vi "Constructor.vi"(11 "Graph Reference":refnum<vi>) -> (3 "Graph Manager out":refnum<class "Graph Manager.lvclass">)   [LabVIEW 2013, in "Graph Manager.lvclass"]
uses:
  Graph Manager.lvclass
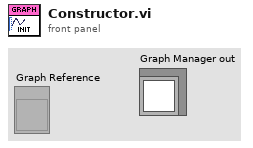
[diagram p1: front panel]
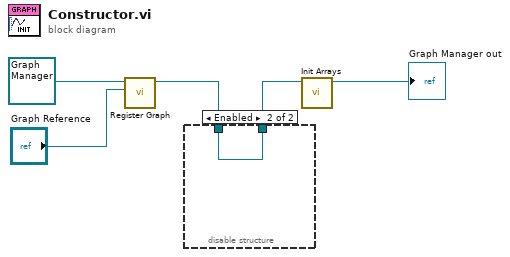
[diagram p0: block diagram]
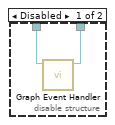
[diagram p2: hidden frame]
diagram:
  n1 = call-dynamic "Register Graph.vi"("Graph Reference"="Graph Reference", "Graph Manager in"=refnum<class "Graph Manager.lvclass"> refnum ("Graph Manager.lvclass")) -> ("Graph Manager out"=w2:refnum<class "Graph Manager.lvclass">)  [unwired: 8 in, 1 out]
  n2 = disable-structure shown="Enabled" {
    disable-tunnel: w2 -> [w7 w8]
    disable-tunnel: [w6 w8] -> w1
    frame Disabled {
      n3 = call "Graph Event Handler.vi"("Graph Manager out 2"=w7) -> ("Graph Manager out"=w6:refnum<class "Graph Manager.lvclass">)  [unwired: 10 in]
    }
    frame Enabled {
    }
  }
  n4 = call-dynamic "Init Arrays.vi"("Graph Manager in"=w1) -> ("Graph Manager out"=→"Graph Manager out":refnum<class "Graph Manager.lvclass">)  [unwired: 9 in, 1 out]
